vi "Actor Core.vi"(8 "error in":errorcluster, 11 "IViewable In":refnum<class "IViewable.lvclass">) -> (0 "error out":errorcluster, 3 "Actor out":refnum<class "Actor.lvclass">)   [LabVIEW 2015, in "IViewable.lvlib" / "IViewable.lvclass"]
doc: "(<B>Filename</B>: Actor Framework.lvlib:Actor.lvclass:Actor Core.vi)\n\nReceives messages to the actor, reacts to them, and initiates any error handling that may shut the actor down.\n\nDescendant classes may override this VI to append parallel tasks for the actor to complete while it handles messages. Overrides use the Call Parent Method node.\n\n<License>\nCopyright © 2017 Composed Systems, LLC | All rights reserved\nwww.composed.io\n\nAuthor: Ethan Stern <ethan.stern@composed.io>\n\nThis software is provided \"AS IS\" WITHOUT WARRANTIES, either express or implied, AND IS FOR EDUCATIONAL PURPOSES ONLY.\n</License>"
uses:
  IViewable.lvclass
  <vilib>/ActorFramework/Actor/Actor.lvclass
  <vilib>/ActorFramework/Actor/Actor.lvclass/Actor.ctl
  <vilib>/ActorFramework/Message Enqueuer/Message Enqueuer.lvclass/Message Enqueuer.ctl
  IViewable.lvclass/IViewable.ctl
  <vilib>/ActorFramework/Message Enqueuer/Init from Existing Queue.vi
  <vilib>/ActorFramework/Message Enqueuer/Enqueue.vi
  <vilib>/ActorFramework/Message Priority Queue/Priority Enqueue.vi
  <vilib>/ActorFramework/Message Enqueuer/Message Enqueuer.lvclass
  IViewable Messages/Resize Panel to Pane Msg/Resize Panel to Pane Msg.lvclass
  AutoRegistration/AutoEventActor/AutoEventActor.lvclass
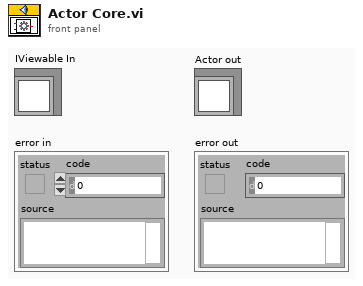
[diagram p1: front panel]
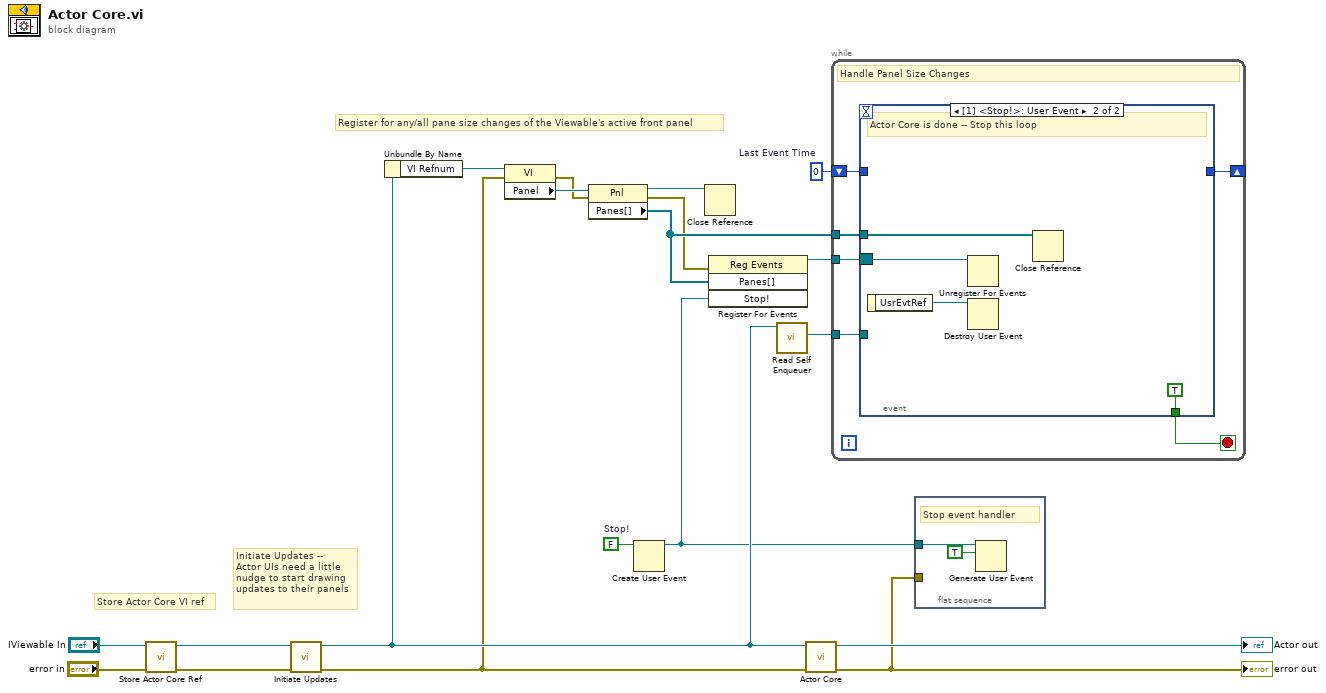
[diagram p0: block diagram]
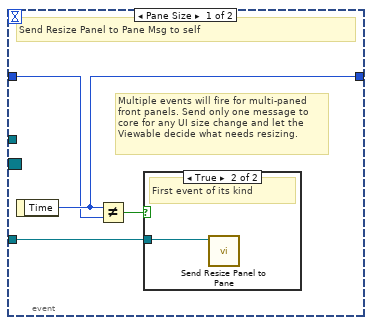
[diagram p2: hidden frame]
diagram:
  w4 = FALSE  # Stop!
  w10 = u32 0  # Last Event Time
  # "Register for any/all pane size changes of the Viewable's active front panel"
  # "Initiate Updates --\nActor UIs need a little\nnudge to start drawing\nupdates to their panels"
  # "Store Actor Core VI ref"
  n1 = call "Store Actor Core Ref.vi"("error in (no error)"="error in", "IViewable In"="IViewable In") -> ("error out"=w13:errorcluster, "IViewable Out"=w12:refnum<class "IViewable.lvclass">)  [unwired: 8 in]
  n2 = call-dynamic "Initiate Updates.vi"("error in (no error)"=w13, "IViewable In"=w12) -> ("error out"=w2:errorcluster, "IViewable Out"=w11:refnum<class "IViewable.lvclass">)  [unwired: 8 in]
  n3 = Unbundle By Name(w11) -> ("VI Refnum"=w5:refnum<vi>)
  n4 = property class="VI"(reference=w5, error in=w2) -> (error out=w7:errorcluster, "Panel"=w8:refnum<vi>)  [unwired: 1 out]
  n5 = property class="Pnl"(reference=w8, error in=w7) -> (reference out=w1:refnum<vi>, error out=w6:errorcluster, "Panes[]"=w14:refnum<vi>[])
  n6 = Create User Event(user event datatype=w4) -> (user event=w3:refnum<user-event>)  [unwired: 1 in, 1 out]
  n7 = Close Reference(reference=w1) -> ()  [unwired: 1 in, 1 out]
  n8 = register-events(error in=w6, w14, w3) -> (reference out=w16:refnum<event-registration>)  [unwired: 1 in, 1 out]
  n9 = call <vilib>:"Read Self Enqueuer.vi"("Actor"=w11) -> ("Self Enqueuer"=w15:refnum<class "Message Enqueuer.lvclass">)  [unwired: 10 in]
  n10 = call-parent "Actor Core.vi"("error in"=w2, "Actor in"=w11) -> ("error out"=w9:errorcluster, "Actor out"=→"Actor out":refnum<class "Actor.lvclass">)  [unwired: 8 in]
  "error out" <- w9
  n11 = while {
    tunnel: w16 -> [w25]
    tunnel: w15 -> [w24]
    tunnel: w14 -> [w22]
    shift-right: [w21] -> _
    shift-left: w10 -> [w20]
    stop <- w23 stop-if-true
    # "Handle Panel Size Changes"
    n12 = event shown="[1] <Stop!>: User Event" {
      selector: w25 -> [_ w32]
      dyn-events: _ -> [_ _]
      timeout: _ -> [_ _]
      tunnel: w24 -> [w26 _]
      tunnel: [_ TRUE] -> w23
      tunnel: w22 -> [_ w33]
      tunnel: [w29 _] -> w21
      tunnel: w20 -> [w28 _]
      event Pane Size {
        # "Multiple events will fire for multi-paned\nfront panels. Send only one message to\ncore for any UI size change and let the\nViewable decide what needs resizing."
        # "Send Resize Panel to Pane Msg to self"
        n13 = event-data() -> ("Time"=w29:u32)  [unwired: 1 in]
        n14 = Not Equal?(x=w29, y=w28) -> (x != y?=w27:bool)
        n15 = case shown="True" w27 {
          tunnel: w26 -> [_ w30]
          frame False {
            # "Flush redundant events"
          }
          frame True {
            # "First event of its kind"
            n16 = call "Send Resize Panel to Pane.vi"("Message Enqueuer"=w30) -> ()  [unwired: 9 in, 2 out]
          }
        }
      }
      event User Event {
        # "Actor Core is done -- Stop this loop"
        n17 = event-data() -> ("UsrEvtRef"=w31:refnum<user-event>)  [unwired: 1 in]
        n18 = Unregister For Events(event registration refnum=w32) -> ()  [unwired: 1 in, 1 out]
        n19 = Destroy User Event(user event=w31) -> ()  [unwired: 1 in, 1 out]
        n20 = Close Reference(reference=w33) -> ()  [unwired: 1 in, 1 out]
      }
    }
  }
  n21 = flat-sequence {
    tunnel: w9 -> [_]
    tunnel: w3 -> [w36]
    frame #0 {
      # "Stop event handler"
      n22 = Generate User Event(user event=w36, event data cluster=TRUE) -> ()  [unwired: 2 in, 2 out]
    }
  }
